vi "LeftClick.vi"(6 "Double Click":bool, 7 "Table History ref":refnum<vi>, 8 "error in (no error)":errorcluster, 9 "Table CtlRef In":refnum<vi>, 10 "Cell Position":T1, 11 "MenuCol in":refnum<class "MenuCol.lvclass">) -> (0 "error out":errorcluster, 1 "Table CtlRef Out":refnum<vi>, 2 "Discard?":bool, 3 "MenuCol out":refnum<class "MenuCol.lvclass">, 5 "Button":u16=1)   [LabVIEW 2013, in "MenuCol.lvclass"]
doc: "For a \"standard\" column, let LabVIEW handle by default. Left-click brings up edit, right-click a shortcut menu. This VI is read only w.r.t the column object."
uses:
  MenuCol.lvclass
  <vilib>/Utility/miscctls.llb/LVRowAndColumnTypeDef.ctl
  TypeDefs/TableHistory.ctl
  TypeDefs/TableArray.ctl
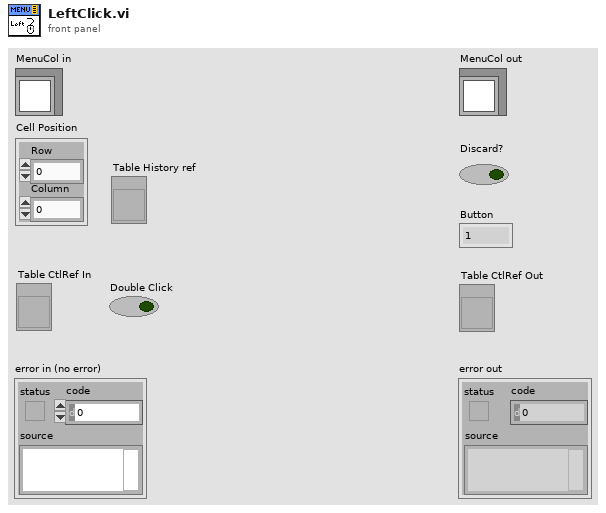
[diagram p1: front panel]
types:
  T1 = typedef "LVRowAndColumnTypeDef.ctl" = cluster{"Row":i32, "Column":i32}
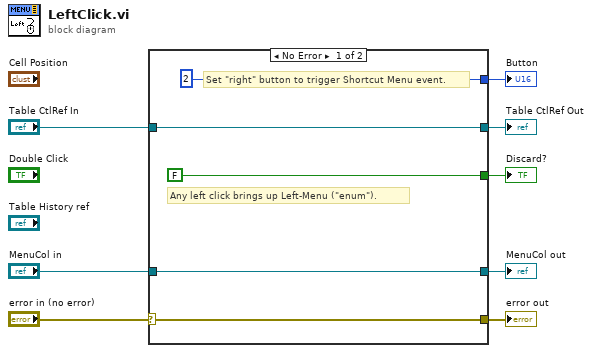
[diagram p0: block diagram]
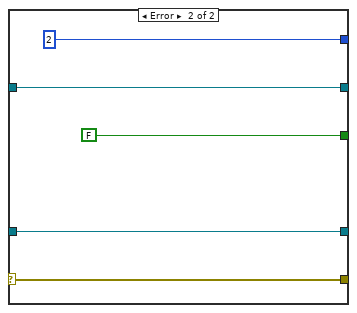
[diagram p2: hidden frame]
diagram:
  n1 = case shown="No Error" "error in (no error)" {
    selector: "error in (no error)" -> [w9 w17]
    tunnel: [FALSE ("Discard?") FALSE ("Discard?")] -> w6
    tunnel: [u16 2 ("Button") u16 2 ("Button")] -> w5
    tunnel: "MenuCol in" -> [w10 w15]
    tunnel: [w10 w15] -> w7
    tunnel: [w9 w17] -> w4
    tunnel: [w11 w18] -> w1
    tunnel: "Table CtlRef In" -> [w11 w18]
    frame No Error {
      # "Set \"right\" button to trigger Shortcut Menu event."
      # "Any left click brings up Left-Menu (\"enum\")."
    }
    frame Error {
    }
  }
  "error out" <- w4
  "MenuCol out" <- w7
  "Discard?" <- w6
  "Table CtlRef Out" <- w1
  "Button" <- w5
